vi "open Subscriber connection.vi"(4 "error in (no error)":errorcluster, 5 "Machine":string="192.168.10.182", 6 "Port":u16=64535, 7 "Subscriber list":string="opticalspectrum") -> (0 "error out":errorcluster, 3 "connection ID":refnum<k5>)   [LabVIEW 2013]
panel:
  out "s? t:f":string
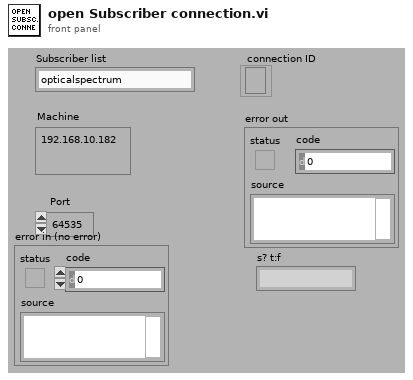
[diagram p1: front panel]
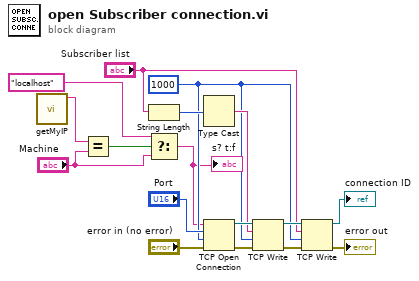
[diagram p0: block diagram]
diagram:
  w6 = 1000 ("timeout ms (60000)")
  n1 = call "getMyIP.vi"() -> ("IP"=w5:string)  [unwired: 11 in]
  n2 = Equal?(x=w5, y="Machine") -> (x = y?=w1:bool)
  n3 = String Length(string="Subscriber list") -> (length=w9:i32)
  n4 = Select(t="localhost" ("IP"), s=w1, f="Machine") -> (s? t:f=w2:string)
  "s? t:f" <- w2
  n5 = Type Cast(x=w9) -> (*(type *) &x=w10:string)  [unwired: 1 in]
  n6 = TCP Open Connection(address=w2, remote port or service name="Port", timeout ms (60000)=w6, error in (no error)="error in (no error)") -> (connection ID=w12:refnum<k5>, error out=w15:errorcluster)  [unwired: 1 out]
  n7 = TCP Write(connection ID=w12, data in=w10, error in (no error)=w15, 9:w6) -> (connection ID out=w13:refnum<k5>, error out=w14:errorcluster)  [unwired: 1 out]
  n8 = TCP Write(connection ID=w13, data in="Subscriber list", error in (no error)=w14, 9:w6) -> (connection ID out=→"connection ID":refnum<k5>, error out=→"error out":errorcluster)  [unwired: 1 out]
